vi "Chirp_DC_Increase.vi"(8 "error in (no error)":errorcluster, 11 "ChirpEIS in":refnum<class "ChirpEIS.lvclass">) -> (0 "error out":errorcluster, 2 "Less than Max DC":bool, 3 "ChirpEIS out":refnum<class "ChirpEIS.lvclass">)   [LabVIEW 2014, in "ChirpEIS.lvclass"]
uses:
  ChirpEIS.lvclass
  ChirpEIS.lvclass/ChirpEIS.ctl
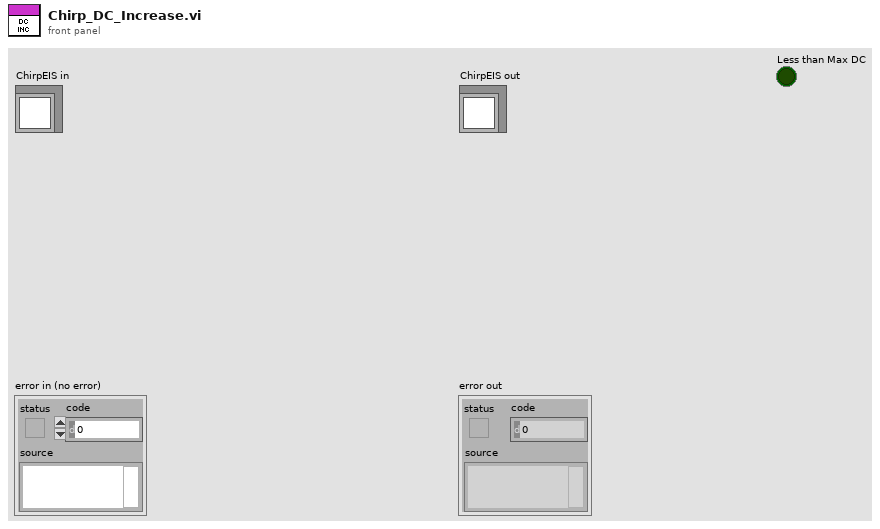
[diagram p1: front panel]
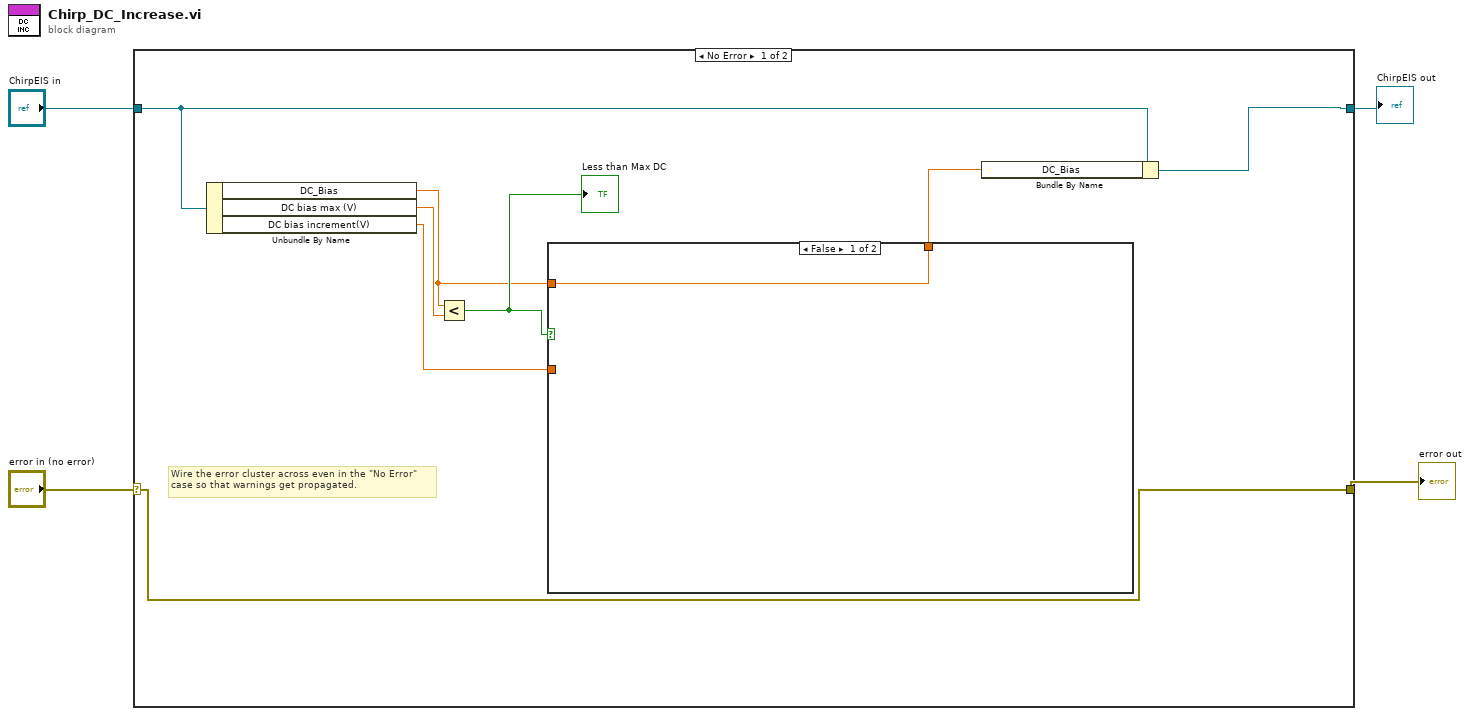
[diagram p0: block diagram]
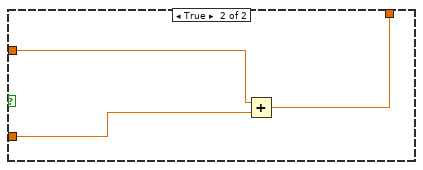
[diagram p2: hidden frame]
diagram:
  n1 = case shown="No Error" "error in (no error)" {
    selector: "error in (no error)" -> [w12 w18]
    tunnel: [w12 w18] -> w3
    tunnel: [w5 w17] -> w1
    tunnel: "ChirpEIS in" -> [w6 w17]
    frame No Error {
      # "Wire the error cluster across even in the \"No Error\"\ncase so that warnings get propagated."
      n2 = Unbundle By Name(w6) -> ("DC_Bias"=w9:dbl, "DC bias max (V)"=w10:dbl, "DC bias increment(V)"=w8:dbl)
      n3 = Less?(x=w9, y=w10) -> (x < y?=w11:bool)
      "Less than Max DC" <- w11
      n4 = case shown="False" w11 {
        tunnel: w9 -> [w13 w16]
        tunnel: [w13 w15] -> w7
        tunnel: w8 -> [_ w14]
        frame False {
        }
        frame True {
          n5 = Add(x=w16, y=w14) -> (x+y=w15:dbl)
        }
      }
      n6 = Bundle By Name(cluster=w6, "DC_Bias"=w7) -> (w5:refnum<class "ChirpEIS.lvclass">)
    }
    frame Error {
    }
  }
  "error out" <- w3
  "ChirpEIS out" <- w1
